vi "hmi_initialize.vi"(7 "hmi_references":T1, 8 "error in (no error)":errorcluster) -> (0 "error out":errorcluster)   [LabVIEW 2015, in "lv-interface-nre.lvlib"]
uses:
  lv-interface-nre.lvlib
  _controls/hmi_references.ctl
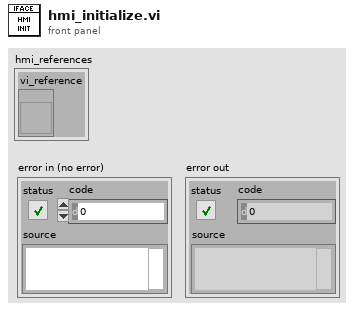
[diagram p1: front panel]
types:
  T1 = typedef "lv-interface-nre.lvlib/hmi_references.ctl" = cluster{"vi_reference":refnum<vi>}
  T2 = enum32{"Invalid", "Standard", "Closed", "Hidden", "Minimized", "Maximized"}
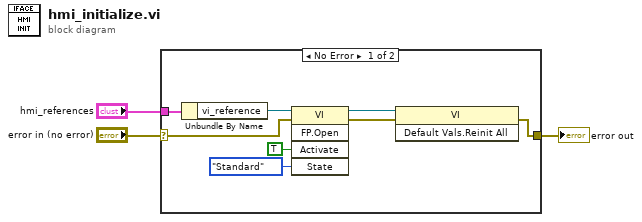
[diagram p0: block diagram]
diagram:
  n1 = case shown="No Error" "error in (no error)" {
    selector: "error in (no error)" -> [w7 w12]
    tunnel: [w4 w12] -> w2
    tunnel: "hmi_references" -> [w8 _]
    frame No Error {
      n2 = Unbundle By Name(w8) -> ("vi_reference"=w11:refnum<vi>)
      n3 = invoke class="VI" method="FP.Open"(reference=w11, error in=w7, "Activate"=TRUE ("Activate?"), "State"=T2."Standard") -> (reference out=w6:refnum<vi>, error out=w5:errorcluster)  [unwired: 1 in, 3 out]
      n4 = invoke class="VI" method="Default Vals.Reinit All"(reference=w6, error in=w5) -> (error out=w4:errorcluster)  [unwired: 1 in, 2 out]
    }
    frame Error {
    }
  }
  "error out" <- w2
